vi "Write LogLevel.vi"(8 "error in (no error)":errorcluster, 10 "LogLevel":T1, 11 "Log Sink in":refnum<class "Log Sink.lvclass">) -> (0 "error out":errorcluster, 3 "Log Sink out":refnum<class "Log Sink.lvclass">)   [LabVIEW 2018, in "MVA Framework.lvlib" / "Composed Log.lvlib" / "Log Sink.lvclass"]
uses:
  Log Sink.lvclass
  Types/Log Level.ctl
  Composed Log.lvlib
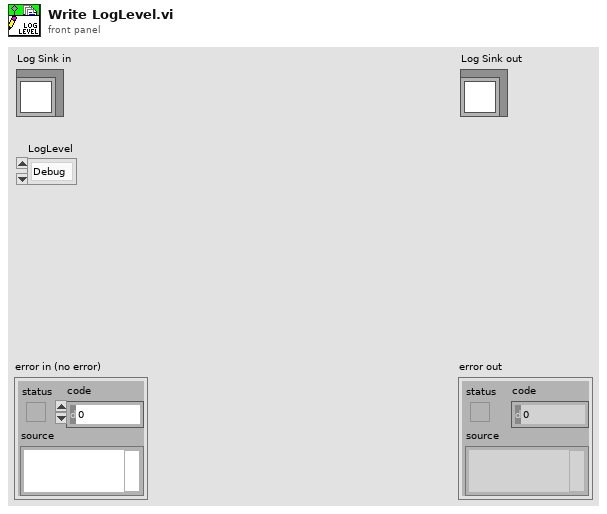
[diagram p1: front panel]
types:
  T1 = typedef "MVA Framework.lvlib/Composed Log.lvlib/Log Level.ctl" = enum16{"Debug", "Info", "Warning", "Error", "Critical"}
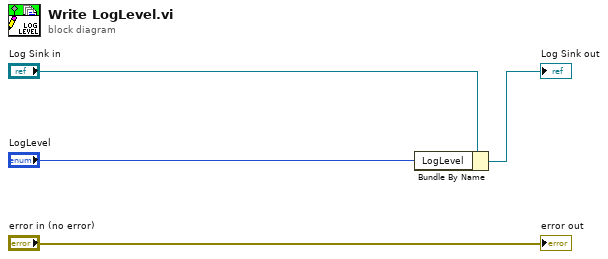
[diagram p0: block diagram]
diagram:
  n1 = Bundle By Name(cluster="Log Sink in", "LogLevel"="LogLevel") -> (→"Log Sink out":refnum<class "Log Sink.lvclass">)
  "error out" <- "error in (no error)"
